vi "Auto Mode FGV.vi"(1 "New Auto Mode":u32, 2 "Action":enum16{"Set", "Get"}(ring)=enum."Get") -> (0 "Auto Mode":u32)   [LabVIEW 2016, in "Huskie Swerve.lvlib"]
uses:
  Huskie Swerve.lvlib
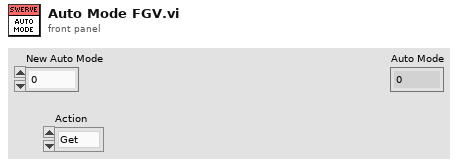
[diagram p1: front panel]
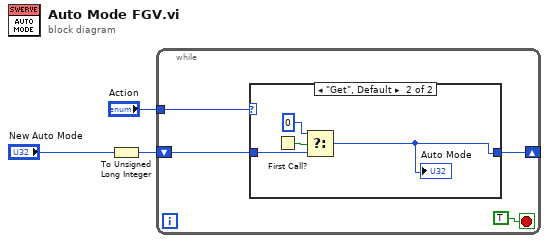
[diagram p0: block diagram]
diagram:
  n1 = To Unsigned Long Integer(number="New Auto Mode") -> (unsigned 32bit integer=w2:u32)
  n2 = while {
    shift-right: [w4] -> _
    shift-left: w2 -> [w5]
    tunnel: "Action" -> [w6]
    stop <- TRUE stop-if-true
    n3 = case shown="\"Get\", Default" w6 {
      tunnel: w5 -> [w8 w10]
      tunnel: [w8 w9] -> w4
      frame "Set" {
      }
      frame "Get", Default {
        n4 = First Call?() -> (First Call?: T/F=w12:bool)
        n5 = Select(t=u32 0, s=w12, f=w10) -> (s? t:f=w9:u32)
        "Auto Mode" <- w9
      }
    }
  }
